vi "Read Raw String.vi"(8 "error in (no error)":errorcluster, 11 "FW Arduino Control in":refnum<class "FW Arduino Control.lvclass">) -> (0 "error out":errorcluster, 2 "Raw String":string, 3 "FW Arduino Control out":refnum<class "FW Arduino Control.lvclass">)   [LabVIEW 2024, in "FW Arduino Control.lvclass"]
uses:
  FW Arduino Control.lvclass
  FW Arduino Control.lvclass/FW Arduino Control.ctl
  Filter Wheel Object/Filter Wheel.lvclass
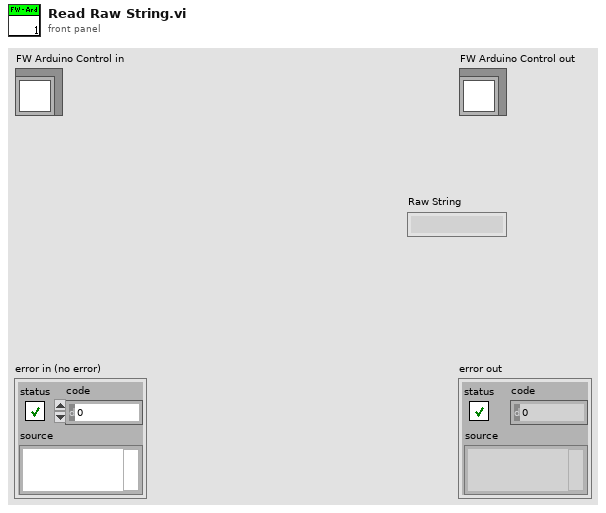
[diagram p1: front panel]
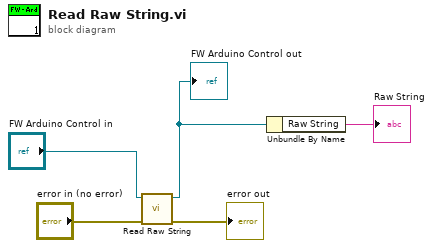
[diagram p0: block diagram]
diagram:
  n1 = call-parent "Read Raw String.vi"("error in (no error)"="error in (no error)", "Filter Wheel in"="FW Arduino Control in") -> ("error out"=→"error out":errorcluster, "Filter Wheel out"=w3:refnum<class "FW Arduino Control.lvclass">)  [unwired: 7 in, 1 out]
  "FW Arduino Control out" <- w3
  n2 = Unbundle By Name(w3) -> ("Raw String"=→"Raw String":string)
